vi "Teleop.vi"(10 "Match Info":T1={"Autonomous Elapsed Seconds"=0.0, "TeleOp Elapsed Seconds"=0.0, "Disabled Elapsed Seconds"=0.0, "Visited Autonomous"=FALSE, "Visited TeleOp"=FALSE, "Visited Disabled"=FALSE, "Autonomous Settings"={"Autonomous Style"=enum."Independent", "VI Refnum"=refnum}}, 11 "Call Context":T2) -> ()   [LabVIEW 2019]
doc: "This VI is called for each TeleOp packet received from the DS where the robot is not disabled. It is often used to read from the joysticks and update I/O or to update setpoints for timed control loops. It should complete and return within 20 milliseconds or it may miss DS packets."
uses:
  <vilib>/Rock Robotics/Network Tables/NT Write Numeric Array.vi
  <vilib>/Rock Robotics/WPI/ThirdParty/Phoenix-LabVIEW/Motor Controller/Controls/CTRE_Phoenix_MotorControl_ControlMode.ctl
  <vilib>/Rock Robotics/Network Tables/NT Write Boolean Array.vi
  <vilib>/Rock Robotics/WPI/RobotDrive/WPI_RobotDriveArcadeDrive_Standard(NoSaturation).vi
  <vilib>/Rock Robotics/WPI/DriverStation/WPI_DriverStationMatch Info.ctl
  <vilib>/Rock Robotics/WPI/DriverStation/WPI_DriverStationDerivedRobotMode.ctl
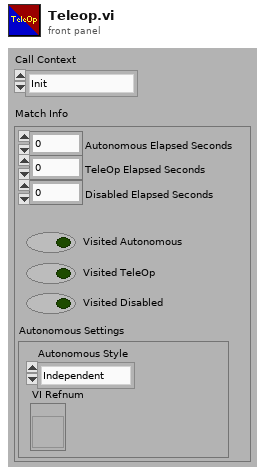
[diagram p1: front panel]
types:
  T1 = typedef "WPI_DriverStationMatch Info.ctl" = cluster{"Autonomous Elapsed Seconds":dbl, "TeleOp Elapsed Seconds":dbl, "Disabled Elapsed Seconds":dbl, "Visited Autonomous":bool, "Visited TeleOp":bool, "Visited Disabled":bool, "Autonomous Settings":cluster{"Autonomous Style":enum16{"Iterative", "Independent"}, "VI Refnum":refnum<vi>}}
  T2 = typedef "WPI_DriverStationDerivedRobotMode.ctl" = enum16{"Init", "Execute", "Stop"}
  T3 = typedef "CTRE_Phoenix_MotorControl_ControlMode.ctl" = u16
  T4 = typedef "WPI_MotorControlDeviceRef.ctl" = cluster{"DeviceStatus":errorcluster, "Type":T5, "PWM":cluster{"PWM Channel":T6, "DeadBand":T7}, "CAN":cluster{"Device Number":u8, "SetOutput VI Ref":variant, "GetOutput VI Ref":variant, "Enable VI Ref":variant, "Disable VI Ref":variant, "Data":variant}, "Invert":bool, "DIO PWM":cluster{"PWM \"Enable\" Channel":T6, "DIOChannel":T8, "PWM Rate":dbl}}
  T5 = typedef "WPI_MotorControlType.ctl" = enum16{"PWM", "CAN", "DIO PWM"}
  T6 = typedef "FPGA_DIOPWMChannel.ctl" = enum8{"PWM 0", "PWM 1", "PWM 2", "PWM 3", "PWM 4", "PWM 5", "PWM 6", "PWM 7", "PWM 8", "PWM 9", "PWM MXP 0", "PWM MXP 1", "PWM MXP 2", "PWM MXP 3", "PWM MXP 4", "PWM MXP 5", "PWM MXP 6", "PWM MXP 7", "PWM MXP 8", "PWM MXP 9", "Invalid"}
  T7 = typedef "WPI_PWMDeadband.ctl" = cluster{"Name":string, "maxPositivePwm":i32, "minPositivePwm":i32, "centerPwm":i32, "maxNegativePwm":i32, "minNegativePwm":i32, "angularRange":u16}
  T8 = typedef "FPGA_DIOChannel.ctl" = enum8{"DIO 0", "DIO 1", "DIO 2", "DIO 3", "DIO 4", "DIO 5", "DIO 6", "DIO 7", "DIO 8", "DIO 9", "DIO MXP 0", "DIO MXP 1", "DIO MXP 2", "DIO MXP 3", "DIO MXP 4", "DIO MXP 5", "DIO MXP 6", "DIO MXP 7", "DIO MXP 8", "DIO MXP 9", "DIO MXP 10", "DIO MXP 11", "DIO MXP 12", "DIO MXP 13", "DIO MXP 14", "DIO MXP 15", "SPI Port CS1", "SPI Port CS2", "SPI Port CS3", "SPI Port MISO", "SPI Port MOSI", "Invalid"}
  T9 = typedef "WPI_JoystickDevRef.ctl" = cluster{"Device":T10}
  T10 = typedef "WPI_JoystickDeviceEnum.ctl" = enum16{"USB 0", "USB 1", "USB 2", "USB 3", "USB 4", "USB 5"}
  T11 = typedef "WPI_RobotDriveDevRef.ctl" = cluster{"DevStatus":errorcluster, "Motors[]":T4[], "Square Inputs":bool, "Max Output":dbl}
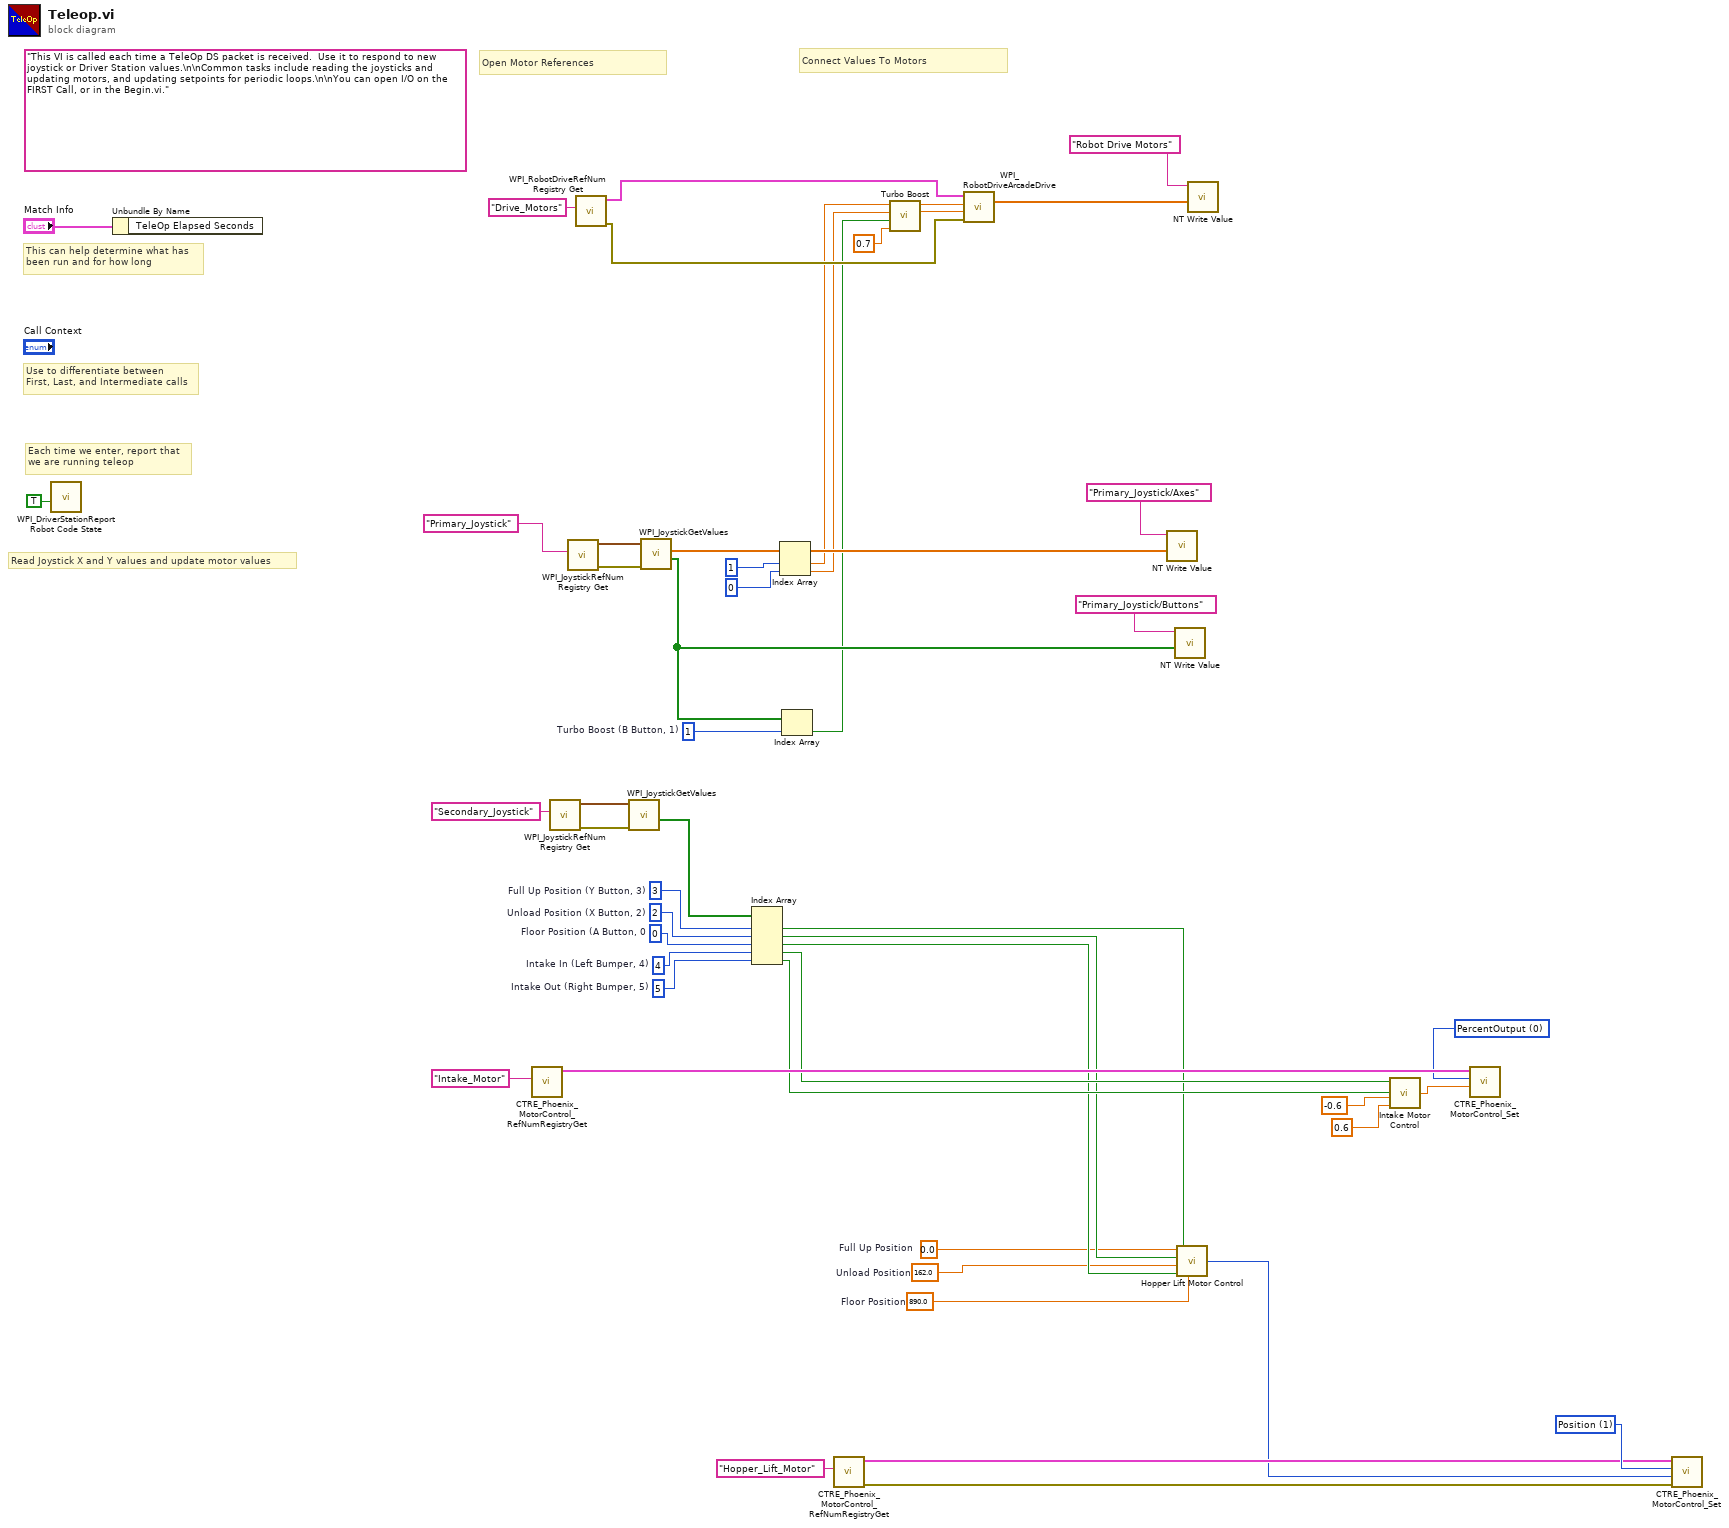
[diagram p0: block diagram]
diagram:
  w1 = 890.0  # Floor Position
  w2 = 162.0  # Unload Position
  w3 = 0.0  # Full Up Position
  w16 = 0  # Floor Position (A Button, 0
  w17 = 2  # Unload Position (X Button, 2)
  w18 = 3  # Full Up Position (Y Button, 3)
  w23 = 5  # Intake Out (Right Bumper, 5)
  w24 = 4  # Intake In (Left Bumper, 4)
  w31 = T3 1 items=["PercentOutput"=0, "Position"=1, "Velocity"=2, "Current"=3, "Follower"=5, "MotionProfile"=6, "MotionMagic"=7, "MotionProfileArc"=10, "Disabled"=15] ("Control Mode")
  w37 = 1  # Turbo Boost (B Button, 1)
  w38 = T3 0 items=["PercentOutput"=0, "Position"=1, "Velocity"=2, "Current"=3, "Follower"=5, "MotionProfile"=6, "MotionMagic"=7, "MotionProfileArc"=10, "Disabled"=15] ("Control Mode")
  (unwired) "This VI is called each time a TeleOp DS packet is received.  Use it to respond to new joystick or Driver Station values.\n\nCommon tasks include reading the joysticks and updating motors, and updating setpoints for periodic loops.\n\nYou can open I/O on the FIRST Call, or in the Begin.vi."
  # "Connect Values To Motors"
  # "Open Motor References"
  # "Each time we enter, report that\nwe are running teleop"
  # "Use to differentiate between\nFirst, Last, and Intermediate calls"
  # "This can help determine what has\nbeen run and for how long"
  # "Read Joystick X and Y values and update motor values"
  n1 = call <vilib>:"WPI_DriverStationReport Robot Code State.vi"("TeleOp"=TRUE ("Autonomous")) -> ()  [unwired: 10 in, 1 out]
  n2 = Unbundle By Name("Match Info") -> ()  [unwired: 1 out]
  n3 = call <vilib>:"CTRE_Phoenix_MotorControl_RefNumRegistryGet.vi"("refnum name"="Intake_Motor") -> ("PhoenixMotorControlDevRef"=w39:T4)  [unwired: 9 in, 1 out]
  n4 = call <vilib>:"WPI_JoystickRefNum Registry Get.vi"("refnum name"="Secondary_Joystick") -> ("error out"=w25:errorcluster, "JoystickDevRef"=w27:T9)  [unwired: 9 in]
  n5 = call <vilib>:"WPI_JoystickRefNum Registry Get.vi"("refnum name"="Primary_Joystick") -> ("error out"=w42:errorcluster, "JoystickDevRef"=w43:T9)  [unwired: 9 in]
  n6 = call <vilib>:"WPI_RobotDriveRefNum Registry Get.vi"("refnum name"="Drive_Motors") -> ("error out"=w47:errorcluster, "RobotDriveDevRef"=w48:T11)  [unwired: 9 in]
  n7 = call <vilib>:"WPI_JoystickGetValues.vi"("error in (no error)"=w25, "JoystickDevRef"=w27) -> ("Buttons"=w22:bool[])  [unwired: 5 in, 4 out]
  n8 = call <vilib>:"WPI_JoystickGetValues.vi"("error in (no error)"=w42, "JoystickDevRef"=w43) -> ("Buttons"=w33:bool[], "Axes"=w36:dbl[])  [unwired: 5 in, 3 out]
  n9 = Index Array(array=w22, index #1=w18, index #2=w17, index #3=w16, index #4=w24, index #5=w23) -> (element #1=w6:bool, element #2=w5:bool, element #3=w4:bool, element #4=w21:bool, element #5=w20:bool)
  n10 = Index Array(array=w36, index #1=1 ("index"), index #2=0 ("index")) -> (element #1=w10:dbl, element #2=w9:dbl)
  n11 = Index Array(array=w33, index=w37) -> (element=w8:bool)
  n12 = call <vilib>:"CTRE_Phoenix_MotorControl_RefNumRegistryGet.vi"("refnum name"="Hopper_Lift_Motor") -> ("error out"=w14:errorcluster, "PhoenixMotorControlDevRef"=w19:T4)  [unwired: 9 in]
  n13 = call "Turbo Boost.vi"("Normal Speed Constant"=0.7, "Turbo Activate Button"=w8, "Y Axis Joystick Input"=w9, "X Axis Joystick Input"=w10) -> ("Y Axis New Value"=w11:dbl, "X Axis New Value"=w12:dbl)  [unwired: 2 in]
  n14 = call-poly <vilib>:"WPI_RobotDriveArcadeDrive.vi"("error in (no error)"=w47, "Y axis value"=w11, "X axis value"=w12, "RobotDriveDevRef"=w48) -> ("Motor Values"=w46:dbl[])  [unwired: 5 in, 2 out]
  n15 = call-poly <vilib>:"NT Write Value.vi"("Numeric Array"=w36, "Name"="Primary_Joystick/Axes") -> ()  [unwired: 9 in, 1 out]
  n16 = call-poly <vilib>:"NT Write Value.vi"("Boolean Array"=w33, "Name"="Primary_Joystick/Buttons") -> ()  [unwired: 9 in, 1 out]
  n17 = call "Hopper Lift Motor Control.vi"("Floor Position"=w1, "Full Up Button"=w6, "Floor Button"=w4, "Unload Position"=w2, "Unload Button"=w5, "Full Up Position"=w3) -> ("New Position"=w15:i32)
  n18 = call-poly <vilib>:"NT Write Value.vi"("Numeric Array"=w46, "Name"="Robot Drive Motors") -> ()  [unwired: 9 in, 1 out]
  n19 = call "Intake Motor Control.vi"("Release Constant"=0.6, "Intake Constant"=-0.6, "Release Button Input"=w20, "Intake Button Input"=w21) -> ("New Scalar"=w28:dbl)
  n20 = call <vilib>:"CTRE_Phoenix_MotorControl_Set.vi"("Output"=w28, "Control Mode"=w38, "PhoenixMotorControlDevRef"=w39) -> ()  [unwired: 7 in, 2 out]
  n21 = call <vilib>:"CTRE_Phoenix_MotorControl_Set.vi"("error in (no error)"=w14, "Output"=w15, "Control Mode"=w31, "PhoenixMotorControlDevRef"=w19) -> ()  [unwired: 6 in, 2 out]
